vi "TDC_getHistogramParams.vi"(8 "Error In":errorcluster) -> (0 "Error Out":errorcluster, 2 "Bin Count":i32, 3 "Bin Width":i32)   [LabVIEW 2011]
uses:
  dist/userlib/lib/tdcbase.dll
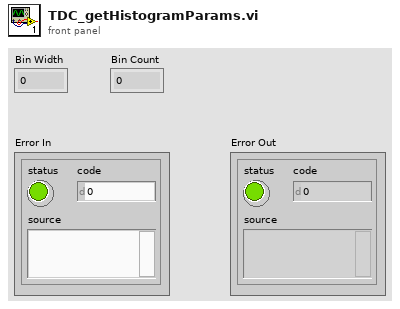
[diagram p1: front panel]
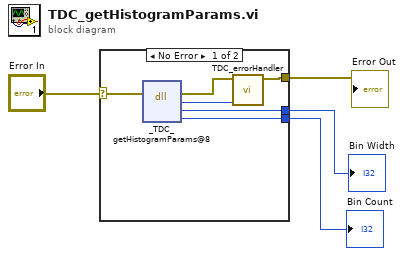
[diagram p0: block diagram]
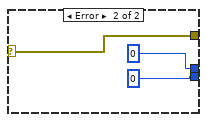
[diagram p2: hidden frame]
diagram:
  n1 = case shown="No Error" "Error In" {
    selector: "Error In" -> [w8 w13]
    tunnel: [w5 w13] -> w3
    tunnel: [w10 0] -> w2
    tunnel: [w9 0] -> w1
    frame No Error {
      n2 = dll-call lib="C:/nh/projekt/spmctrl/dist/userlib/lib/tdcbase.dll" fn="_TDC_getHistogramParams@8"(error in=w8) -> (error out=w7:errorcluster, "return type"=w6:i32, "binWidth"=w10:i32, "binCount"=w9:i32)  [unwired: 4 in, 1 out]
      n3 = call "TDC_errorHandler.vi"("quTAU Return Code"=w6, "Error In"=w7) -> ("Error Out"=w5:errorcluster)  [unwired: 9 in]
    }
    frame Error {
    }
  }
  "Error Out" <- w3
  "Bin Width" <- w2
  "Bin Count" <- w1
